vi "Post-Install Custom Action.vi"(10 "Variant":variant) -> (0 "error out":errorcluster)   [LabVIEW 2013]
panel:
  out "error out 2":errorcluster
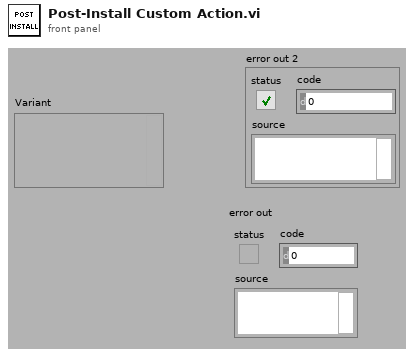
[diagram p1: front panel]
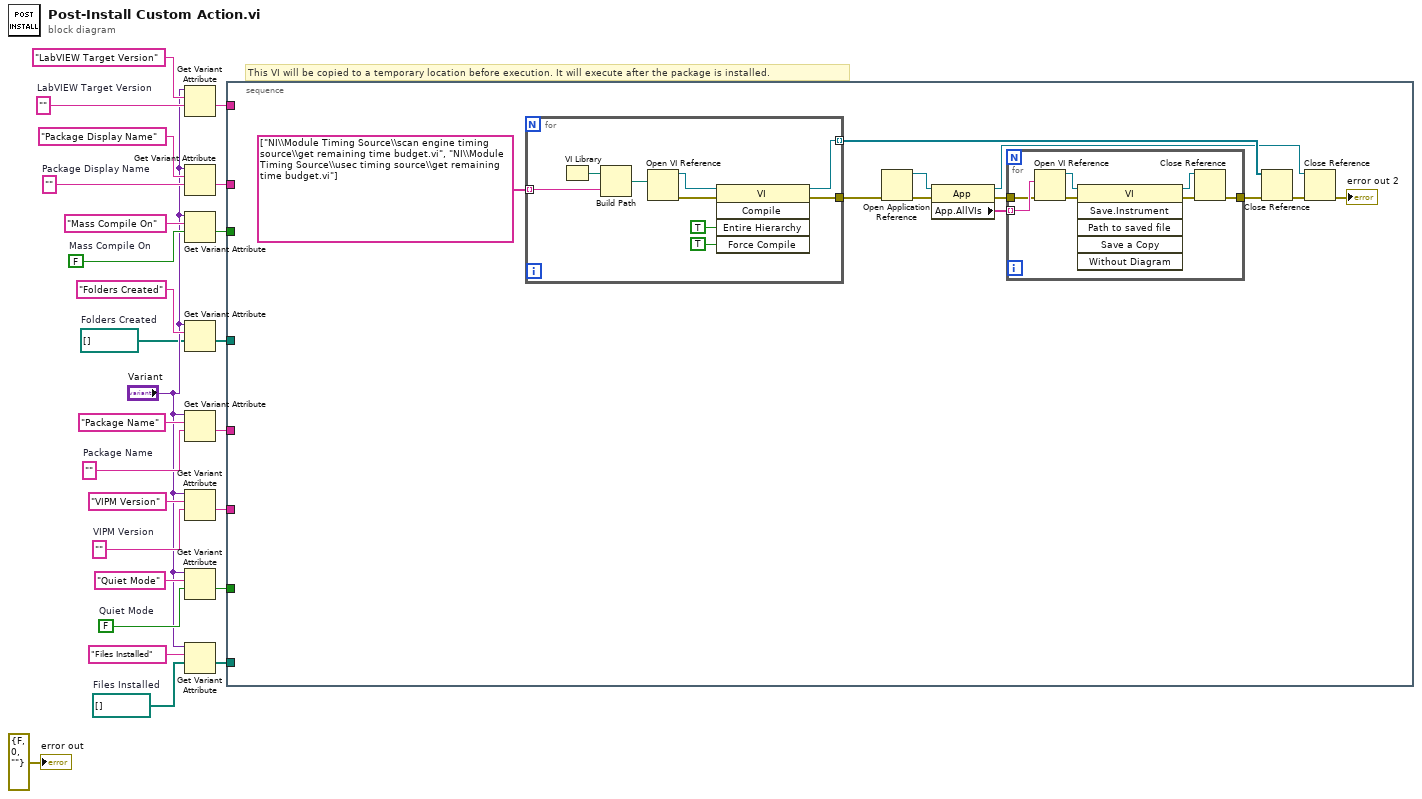
[diagram p0: block diagram]
diagram:
  w1 = path[] []  # Folders Created
  w2 = path[] []  # Files Installed
  w8 = FALSE  # Mass Compile On
  w9 = ""  # Package Display Name
  w16 = FALSE  # Quiet Mode
  w19 = ""  # VIPM Version
  w21 = ""  # LabVIEW Target Version
  w23 = ""  # Package Name
  # "This VI will be copied to a temporary location before execution. It will execute after the package is installed."
  n1 = Get Variant Attribute(Variant="Variant", name="LabVIEW Target Version", default value (empty Variant)=w21) -> (value=w13:string)  [unwired: 1 in, 3 out]
  n2 = Get Variant Attribute(Variant="Variant", name="Package Display Name", default value (empty Variant)=w9) -> (value=w15:string)  [unwired: 1 in, 3 out]
  n3 = Get Variant Attribute(Variant="Variant", name="Mass Compile On", default value (empty Variant)=w8) -> (value=w10:bool)  [unwired: 1 in, 3 out]
  n4 = Get Variant Attribute(Variant="Variant", name="Folders Created", default value (empty Variant)=w1) -> (value=w6:path[])  [unwired: 1 in, 3 out]
  n5 = Get Variant Attribute(Variant="Variant", name="Package Name", default value (empty Variant)=w23) -> (value=w14:string)  [unwired: 1 in, 3 out]
  n6 = Get Variant Attribute(Variant="Variant", name="VIPM Version", default value (empty Variant)=w19) -> (value=w12:string)  [unwired: 1 in, 3 out]
  n7 = Get Variant Attribute(Variant="Variant", name="Quiet Mode", default value (empty Variant)=w16) -> (value=w11:bool)  [unwired: 1 in, 3 out]
  n8 = Get Variant Attribute(Variant="Variant", name="Files Installed", default value (empty Variant)=w2) -> (value=w5:path[])  [unwired: 1 in, 3 out]
  n9 = stacked-sequence {
    tunnel: w15 -> [_]
    tunnel: w14 -> [_]
    tunnel: w13 -> [_]
    tunnel: w12 -> [_]
    tunnel: w11 -> [_]
    tunnel: w10 -> [_]
    tunnel: w5 -> [_]
    tunnel: w6 -> [_]
    frame #0 {
      n10 = for {
        tunnel: [w42] -> w37
        tunnel: [w41] -> w32 mode=indexing
        tunnel: string[] ["NI\\Module Timing Source\\scan engine timing source\\get remaining time budget.vi", "NI\\Module Timing Source\\usec timing source\\get remaining time budget.vi"] -> [w38] mode=indexing
        n11 = VI Library() -> (path=w40:path)
        n12 = Build Path(base path=w40, name or relative path=w38) -> (appended path=w39:path)
        n13 = Open VI Reference(vi path=w39) -> (vi reference=w46:refnum<vi>, error out=w45:errorcluster)  [unwired: 5 in]
        n14 = invoke class="VI" method="Compile"(reference=w46, error in=w45, "Entire Hierarchy"=TRUE ("Compile Entire Hierarchy (F)"), "Force Compile"=TRUE ("Force Compile (T)")) -> (reference out=w41:refnum<vi>, error out=w42:errorcluster)  [unwired: 1 in, 3 out]
      }
      n15 = Open Application Reference(8:w37) -> (0:w34:errorcluster, 3:w36:refnum<vi>)  [unwired: 3 in]
      n16 = property class="App"(reference=w36, error in=w34) -> (reference out=w30:refnum<vi>, error out=w28:errorcluster, "App.AllVIs"=w35:string[])
      n17 = for {
        tunnel: w35 -> [w53] mode=indexing
        tunnel: [w48] -> w33
        tunnel: w28 -> [w47]
        n18 = Open VI Reference(vi path=w53, error in (no error)=w47) -> (vi reference=w52:refnum<vi>, error out=w51:errorcluster)  [unwired: 4 in]
        n19 = invoke class="VI" method="Save.Instrument"(reference=w52, error in=w51) -> (reference out=w50:refnum<vi>, error out=w49:errorcluster)  [unwired: 4 in, 4 out]
        n20 = Close Reference(reference=w50, error in (no error)=w49) -> (error out=w48:errorcluster)
      }
      n21 = Close Reference(reference=w32, error in (no error)=w33) -> (error out=w31:errorcluster)
      n22 = Close Reference(reference=w30, error in (no error)=w31) -> (error out=→"error out 2":errorcluster)
    }
  }
  "error out" <- errorcluster {"status"=FALSE, "code"=0, "source"=""} ("error out")
